vi "Slide Control  Position.vi"(6 "Direction":enum16{"Right", "Left", "Down", "Up"}(ring), 8 "error in":errorcluster, 11 "Ctl Refnum":refnum<vi>) -> (0 "error out":errorcluster)   [LabVIEW 2016]
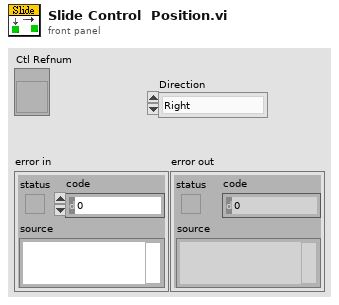
[diagram p1: front panel]
types:
  T1 = typedef "LVPositionTypeDef.ctl" = cluster{"Left":i32, "Top":i32}
  T2 = typedef "LVBoundsTypeDef.ctl" = cluster{"Width":u32, "Height":u32}
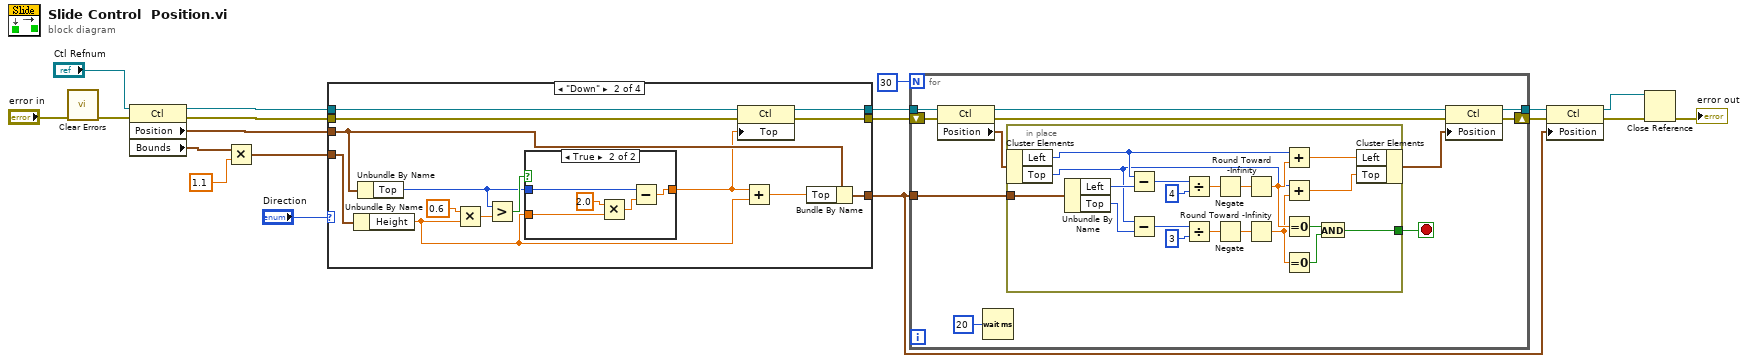
[diagram p0: block diagram]
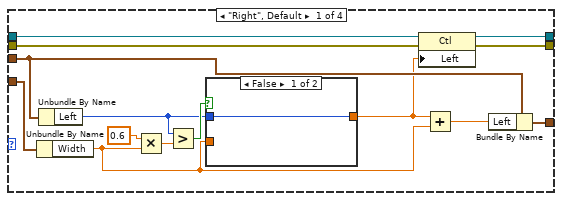
[diagram p2: hidden frame]
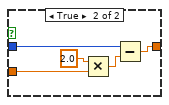
[diagram p3: hidden frame]
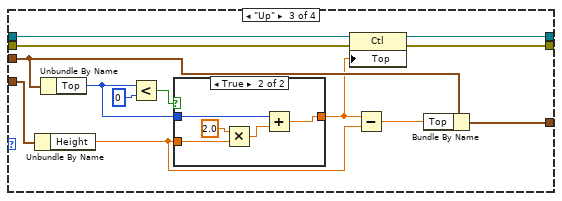
[diagram p5: hidden frame]
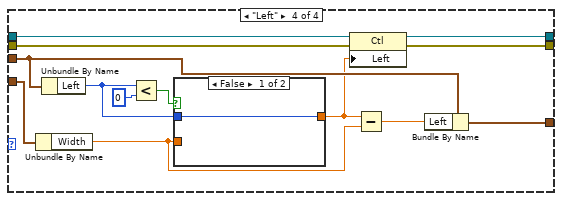
[diagram p7: hidden frame]
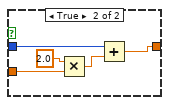
[diagram p8: hidden frame]
diagram:
  n1 = call <vilib>:"Clear Errors.vi"("error in (no error)"="error in") -> ("error out"=w2:errorcluster)  [unwired: 5 in, 1 out]
  n2 = property on="Property Node" class="Ctl"(reference="Ctl Refnum", error in=w2) -> (reference out=w12:refnum<vi>, error out=w10:errorcluster, "Position"=w17:T1, "Bounds"=w15:T2)
  n3 = Multiply(x=w15, y=1.1) -> (x*y=w14:cluster{"Width":dbl, "Height":dbl})
  n4 = case shown="\"Down\"" "Direction" {
    tunnel: w17 -> [w27 w47 w66 w85]
    tunnel: w14 -> [w33 w53 w72 w91]
    tunnel: [w32 w52 w71 w90] -> w13
    tunnel: w12 -> [w31 w51 w70 w89]
    tunnel: [w30 w50 w69 w88] -> w11
    tunnel: w10 -> [w29 w49 w68 w87]
    tunnel: [w28 w48 w67 w86] -> w9
    frame "Right", Default {
      n5 = Unbundle By Name(w33) -> ("Width"=w23:dbl)
      n6 = Unbundle By Name(w27) -> ("Left"=w22:i32)
      n7 = Multiply(x=0.6, y=w23) -> (x*y=w26:dbl)
      n8 = Greater?(x=w22, y=w26) -> (0:w24:bool)
      n9 = case shown="False" w24 {
        tunnel: w23 -> [_ w37]
        tunnel: w22 -> [w34 w36]
        tunnel: [w34 w35] -> w21
        frame False {
        }
        frame True {
          n10 = Multiply(x=2.0 ("y"), y=w37) -> (x*y=w39:dbl)
          n11 = Subtract(x=w36, y=w39) -> (x-y=w35:dbl)
        }
      }
      n12 = property on="Property Node" class="Ctl"(reference=w31, error in=w29, "Left"=w21) -> (reference out=w30:refnum<vi>, error out=w28:errorcluster)
      n13 = Add(x=w21, y=w23) -> (x+y=w20:dbl)
      n14 = Bundle By Name(cluster=w27, "Left"=w20) -> (w32:T1)
    }
    frame "Down" {
      n15 = Unbundle By Name(w53) -> ("Height"=w43:dbl)
      n16 = Unbundle By Name(w47) -> ("Top"=w42:i32)
      n17 = Multiply(x=0.6, y=w43) -> (x*y=w46:dbl)
      n18 = Greater?(x=w42, y=w46) -> (0:w44:bool)
      n19 = case shown="True" w44 {
        tunnel: w43 -> [_ w57]
        tunnel: w42 -> [w54 w56]
        tunnel: [w54 w55] -> w40
        frame False {
        }
        frame True {
          n20 = Multiply(x=2.0 ("y"), y=w57) -> (x*y=w59:dbl)
          n21 = Subtract(x=w56, y=w59) -> (x-y=w55:dbl)
        }
      }
      n22 = property on="Property Node" class="Ctl"(reference=w51, error in=w49, "Top"=w40) -> (reference out=w50:refnum<vi>, error out=w48:errorcluster)
      n23 = Add(x=w40, y=w43) -> (x+y=w41:dbl)
      n24 = Bundle By Name(cluster=w47, "Top"=w41) -> (w52:T1)
    }
    frame "Up" {
      n25 = Unbundle By Name(w72) -> ("Height"=w64:dbl)
      n26 = Unbundle By Name(w66) -> ("Top"=w62:i32)
      n27 = Less?(x=w62, y=0 ("x")) -> (x < y?=w65:bool)
      n28 = case shown="True" w65 {
        tunnel: w64 -> [_ w76]
        tunnel: w62 -> [w73 w75]
        tunnel: [w73 w74] -> w60
        frame False {
        }
        frame True {
          n29 = Multiply(x=2.0 ("y"), y=w76) -> (x*y=w78:dbl)
          n30 = Add(x=w75, y=w78) -> (x+y=w74:dbl)
        }
      }
      n31 = property on="Property Node" class="Ctl"(reference=w70, error in=w68, "Top"=w60) -> (reference out=w69:refnum<vi>, error out=w67:errorcluster)
      n32 = Subtract(x=w60, y=w64) -> (x-y=w61:dbl)
      n33 = Bundle By Name(cluster=w66, "Top"=w61) -> (w71:T1)
    }
    frame "Left" {
      n34 = Unbundle By Name(w91) -> ("Width"=w83:dbl)
      n35 = Unbundle By Name(w85) -> ("Left"=w81:i32)
      n36 = Less?(x=w81, y=0 ("x")) -> (x < y?=w84:bool)
      n37 = case shown="False" w84 {
        tunnel: w83 -> [_ w95]
        tunnel: w81 -> [w92 w94]
        tunnel: [w92 w93] -> w79
        frame False {
        }
        frame True {
          n38 = Multiply(x=2.0 ("y"), y=w95) -> (x*y=w97:dbl)
          n39 = Add(x=w94, y=w97) -> (x+y=w93:dbl)
        }
      }
      n40 = property on="Property Node" class="Ctl"(reference=w89, error in=w87, "Left"=w79) -> (reference out=w88:refnum<vi>, error out=w86:errorcluster)
      n41 = Subtract(x=w79, y=w83) -> (x-y=w80:dbl)
      n42 = Bundle By Name(cluster=w85, "Left"=w80) -> (w90:T1)
    }
  }
  n43 = for {
    N: 30 -> [_]
    tunnel: w11 -> [w105]
    shift-right: [w102] -> w6
    shift-left: w9 -> [w104]
    tunnel: [w100] -> w7
    tunnel: w13 -> [w99]
    stop <- w101 stop-if-true
    n44 = property on="Property Node" class="Ctl"(reference=w105, error in=w104) -> (reference out=w98:refnum<vi>, error out=w103:errorcluster, "Position"=w108:T1)
    n45 = Wait (ms)(milliseconds to wait=u32 20) -> ()  [unwired: 1 out]
    n46 = in-place {
      in-place-border: [w118] -> w101
      in-place-border: w99 -> [w117]
      n47 = in-place-cluster #1(w108) -> ("Left"=w126:i32, "Top"=w114:i32)
      n48 = Unbundle By Name(w117) -> ("Left"=w116:i32, "Top"=w115:i32)
      n49 = Subtract(x=w126, y=w116) -> (x-y=w128:i32)
      n50 = Subtract(x=w114, y=w115) -> (x-y=w124:i32)
      n51 = Divide(x=w128, y=4) -> (x/y=w112:dbl)
      n52 = Divide(x=w124, y=3) -> (x/y=w111:dbl)
      n53 = Negate(x=w112) -> (-x=w110:dbl)
      n54 = Negate(x=w111) -> (-x=w109:dbl)
      n55 = Round Toward -Infinity(1:w110) -> (0:w127:dbl)
      n56 = Round Toward -Infinity(1:w109) -> (0:w125:dbl)
      n57 = Add(x=w126, y=w127) -> (x+y=w113:dbl)
      n58 = Add(x=w114, y=w125) -> (x+y=w121:dbl)
      n59 = Equal To 0?(x=w127) -> (x = 0?=w119:bool)
      n60 = Equal To 0?(x=w125) -> (x = 0?=w120:bool)
      n61 = And(x=w119, y=w120) -> (x .and. y?=w118:bool)
      n62 = in-place-cluster #1("Left"=w113, "Top"=w121) -> (w107:T1)
    }
    n63 = property on="Property Node" class="Ctl"(reference=w98, error in=w103, "Position"=w107) -> (reference out=w100:refnum<vi>, error out=w102:errorcluster)
  }
  n64 = property on="Property Node" class="Ctl"(reference=w7, error in=w6, "Position"=w13) -> (reference out=w4:refnum<vi>, error out=w5:errorcluster)
  n65 = Close Reference(reference=w4, error in (no error)=w5) -> (error out=→"error out":errorcluster)
